vi "Page_Info_Validate_Filename.vi"(8 "error in (no error)":errorcluster, 10 "Filename in":string, 11 "AB_DepDLL in":refnum<class "AB_DepDLL.lvclass">) -> (0 "error out":errorcluster, 1 "hasInvalidCharacters":bool, 2 "Filename out":string, 3 "AB_DepDLL out":refnum<class "AB_DepDLL.lvclass">, 5 "message":string)   [LabVIEW 2020, in "AB_DepDLL.lvclass"]
uses:
  <vilib>/AppBuilder/AB_Classes/DepDLL/AB_DepDLL.lvclass
  e:/builds/penguin/labview/branches/2020/dev/dist/vi.lib/AppBuilder/AB_Classes/Build/AB_Build.lvclass
  <vilib>/AppBuilder/AB_Classes/DLL/AB_DLL.lvclass
  <vilib>/AppBuilder/AB_Classes/Deployment/AB_Deployment.lvlib
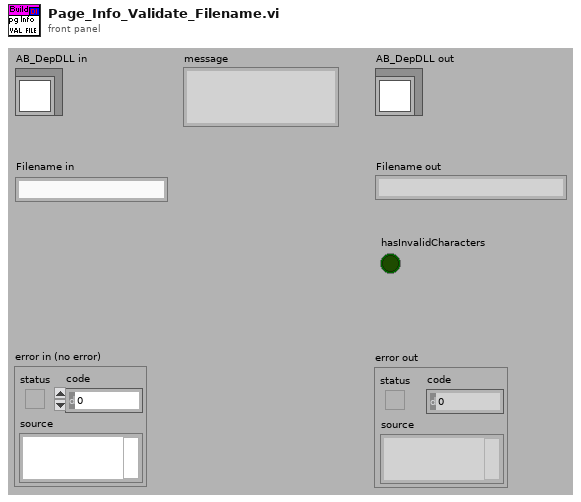
[diagram p1: front panel]
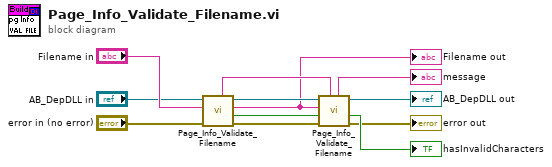
[diagram p0: block diagram]
diagram:
  n1 = call-parent <vilib>:"Page_Info_Validate_Filename.vi"("error in (no error)"="error in (no error)", "Filename in"="Filename in", "AB_DLL in"="AB_DepDLL in") -> ("error out"=w8:errorcluster, "hasInvalidCharacters"=w10:bool, "Filename out"=w1:string, "AB_DLL out"=w4:refnum<class "AB_DepDLL.lvclass">, "message"=w2:string)  [unwired: 4 in]
  "Filename out" <- w1
  n2 = call <vilib>:"Page_Info_Validate_Filename.vi"("message"=w2, "error in (no error)"=w8, "hasInvalidCharacters"=w10, "Filename"=w1, "Build in"=w4) -> ("error out"=→"error out":errorcluster, "hasInvalidCharacters"=→"hasInvalidCharacters":bool, "Build out"=→"AB_DepDLL out":refnum<class "AB_DepDLL.lvclass">, "message"=→"message":string)  [unwired: 3 in]
